vi "图形控件之三维图形的使用.vi"() -> ()   [LabVIEW 2018]
uses:
  <vilib>/Math Plots/3D Math Plots/3D Surface/3D Surface XCtrl/3D Surface.xctl
  <vilib>/Math Plots/3D Math Plots/3D Contour/3D Contour XCtrl/3D Contour.xctl
  <vilib>/Math Plots/3D Math Plots/3D Pie/3D Pie XCtrl/3D Pie.xctl
  <vilib>/Math Plots/3D Math Plots/3D Surface/3D Surface Datatype/Public/Plot Helper (Vector).vi
  <vilib>/Math Plots/3D Math Plots/3D Contour/3D Contour Datatype/Public/Plot Helper (Vector).vi
  <vilib>/Math Plots/3D Math Plots/3D Pie/3D Pie Datatype/Public/Plot Helper (Vector).vi
  <vilib>/Math Plots/3D Math Plots/3D Surface/3D Surface Datatype/3D Surface Datatype.lvclass
  <vilib>/Math Plots/3D Math Plots/3D Contour/3D Contour Datatype/3D Contour Datatype.lvclass
  <vilib>/Math Plots/3D Math Plots/3D Pie/3D Pie Datatype/3D Pie Datatype.lvclass
panel:
  in  "数组 2":dbl[](array[numeric])
  in  "数组":dbl[](array[numeric])
  out "3D Pie":refnum<class "3D Plot Datatype.lvclass">[](xcontrol) caption="三维饼图"
  out "3D Contour":refnum<class "3D Plot Datatype.lvclass">[](xcontrol) caption="三维等高线"
  out "3D Surface":refnum<class "3D Plot Datatype.lvclass">[](xcontrol) caption="三维曲面"
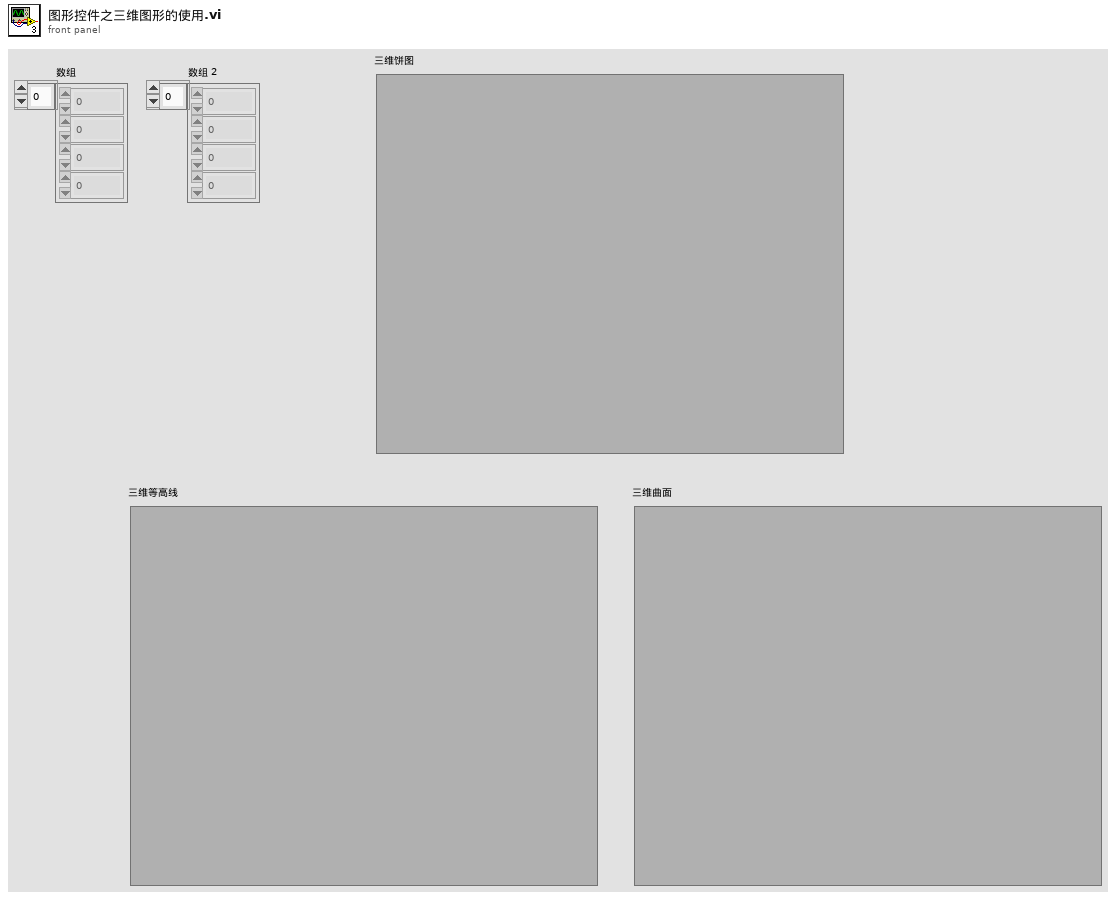
[diagram p1: front panel]
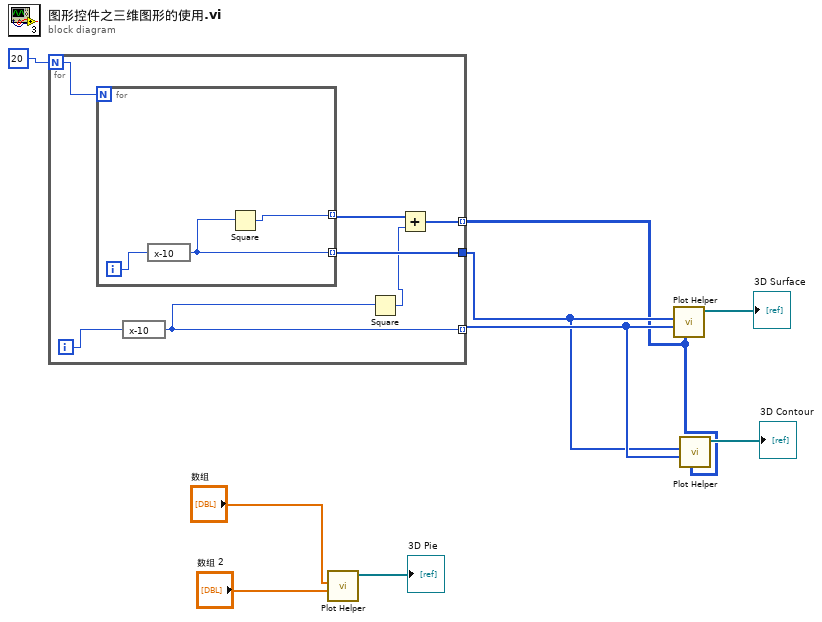
[diagram p0: block diagram]
diagram:
  n1 = for {
    N: 20 -> [w16]
    tunnel: [w13] -> w6 mode=indexing
    tunnel: [w14] -> w5
    tunnel: [w10] -> w4 mode=indexing
    i -> [w15]
    n2 = for {
      N: w16 -> [_]
      tunnel: [w18] -> w14 mode=indexing
      tunnel: [w17] -> w11 mode=indexing
      i -> [w19]
      n3 = expression code="x-10"(w19) -> (w18:i32)
      n4 = Square(x=w18) -> (x^2=w17:i32)
    }
    n5 = expression code="x-10"(w15) -> (w13:i32)
    n6 = Square(x=w13) -> (x^2=w12:i32)
    n7 = Add(x=w11, y=w12) -> (x+y=w10:i32[])
  }
  n8 = call-poly <vilib>:"Plot Helper.vi"("offset vector"="数组 2", "x vector"="数组") -> ("3D Plot lvclass Array out"=→"3D Pie":refnum<class "3D Plot Datatype.lvclass">[])  [unwired: 1 in, 8 out]
  n9 = call-poly <vilib>:"Plot Helper.vi"("z matrix"=w4, "y vector"=w6, "x vector"=w5) -> ("3D Plot lvclass Array out"=→"3D Surface":refnum<class "3D Plot Datatype.lvclass">[])  [unwired: 3 in, 5 out]
  n10 = call-poly <vilib>:"Plot Helper.vi"("z matrix"=w4, "y vector"=w6, "x vector"=w5) -> ("3D Plot lvclass Array out"=→"3D Contour":refnum<class "3D Plot Datatype.lvclass">[])  [unwired: 3 in, 5 out]
